vi "ROI from INI Section.vi"(7 "section":string="Parameters", 8 "error in (no error)":errorcluster, 11 "refnum in":T1) -> (0 "error out":errorcluster, 2 "ROI":T2 {"Contours"."Type" items=["No Selection", "Point", "Line", "Rectangle", "Oval", "Polygon", "Freehand Region", "Annulus", "Unused2", "Unused3", "Broken Line", "Freehand Line", "Rotated Rectangle"]}, 3 "refnum out":T1)   [LabVIEW 2020, in "POLARIS Vision utility.lvlib"]
uses:
  POLARIS Vision utility.lvlib
  <vilib>/Utility/config.llb/Config Data RefNum.ctl
  <vilib>/Utility/config.llb/Read Key (I32).vi
  <vilib>/Utility/config.llb/NI_LVConfig.lvlib
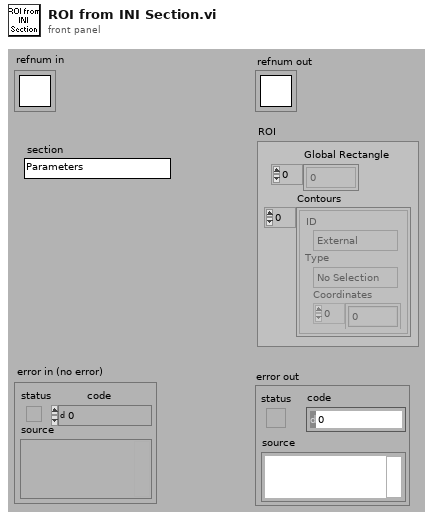
[diagram p1: front panel]
types:
  T1 = typedef "NI_LVConfig.lvlib/Config Data RefNum.ctl" = refnum<k1>
  T2 = typedef "ROI Descriptor" = cluster{"Global Rectangle":i32[], "Contours":cluster{"ID":enum32{"External", "Internal"}, "Type":u32, "Coordinates":i32[]}[]}
  T3 = cluster{"ID":enum32{"External", "Internal"}, "Type":u32, "Coordinates":i32[]}[]
  T4 = cluster{"ID":enum32{"External", "Internal"}, "Type":u32, "Coordinates":i32[]}
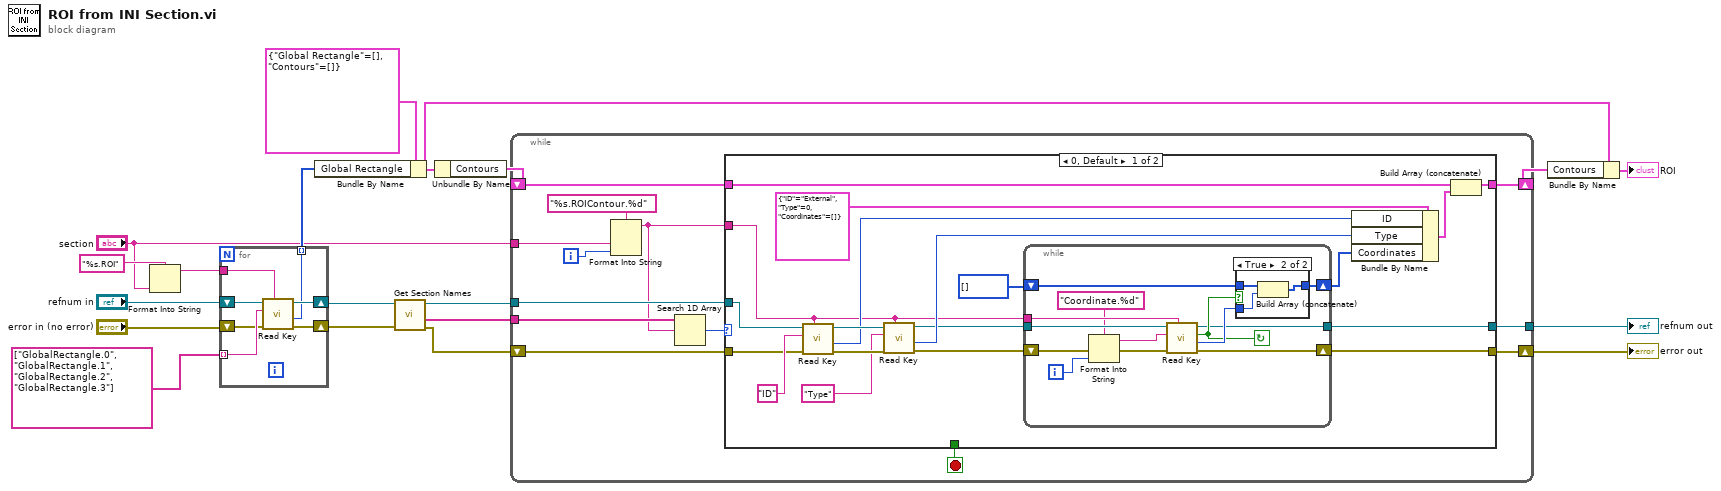
[diagram p0: block diagram]
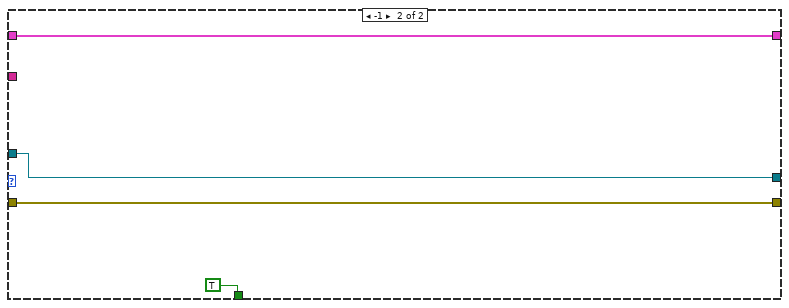
[diagram p3: hidden frame]
diagram:
  n1 = Format Into String(format string="%s.ROI", "section") -> (resulting string=w2:string)  [unwired: 2 in, 1 out]
  n2 = for {
    tunnel: string[] ["GlobalRectangle.0", "GlobalRectangle.1", "GlobalRectangle.2", "GlobalRectangle.3"] -> [w25] mode=indexing
    shift-right: [w24] -> w6
    shift-left: "refnum in" -> [w26]
    shift-right: [w22] -> w7
    shift-left: "error in (no error)" -> [w23]
    tunnel: [w21] -> w14 mode=indexing
    tunnel: w2 -> [w20]
    n3 = call-poly <vilib>:"Read Key.vi"("section"=w20, "error in (no error)"=w23, "key"=w25, "refnum"=w26) -> ("error out"=w22:errorcluster, "value"=w21:i32, "refnum out"=w24:T1)  [unwired: 4 in, 1 out]
  }
  n4 = Bundle By Name(cluster=T2 {"Global Rectangle"=[], "Contours"=[]} ("ROI Descriptor"), "Global Rectangle"=w14) -> (w12:T2)
  n5 = call <vilib>:"Get Section Names.vi"("error in (no error)"=w7, "refnum"=w6) -> ("error out"=w4:errorcluster, "section names"=w13:string[], "refnum out"=w5:T1)  [unwired: 7 in]
  n6 = Unbundle By Name(w12) -> ("Contours"=w17:T3)
  n7 = while {
    tunnel: w13 -> [w38]
    tunnel: w5 -> [w35]
    shift-right: [w33] -> w18
    shift-left: w4 -> [w34]
    tunnel: [w32] -> w19
    shift-right: [w30] -> w11
    shift-left: w17 -> [w31]
    tunnel: "section" -> [w28]
    i -> [w29]
    stop <- w36 stop-if-true
    n8 = Format Into String(format string="%s.ROIContour.%d" ("section"), w28, w29) -> (resulting string=w27:string)  [unwired: 2 in, 1 out]
    n9 = Search 1D Array(1D array=w38, element=w27) -> (index of element=w37:i32)  [unwired: 1 in]
    n10 = case shown="0, Default" w37 {
      tunnel: [_ TRUE] -> w36
      tunnel: w27 -> [w47 _]
      tunnel: w35 -> [w57 w77]
      tunnel: w34 -> [w56 w78]
      tunnel: w31 -> [w41 w76]
      tunnel: [w45 w78] -> w33
      tunnel: [w44 w77] -> w32
      tunnel: [w40 w76] -> w30
      frame 0, Default {
        n11 = call-poly <vilib>:"Read Key.vi"("section"=w47, "error in (no error)"=w56, "key"="ID", "refnum"=w57) -> ("error out"=w55:errorcluster, "value"=w51:i32, "refnum out"=w54:T1)  [unwired: 4 in, 1 out]
        n12 = call-poly <vilib>:"Read Key.vi"("section"=w47, "error in (no error)"=w55, "key"="Type", "refnum"=w54) -> ("error out"=w49:errorcluster, "value"=w50:i32, "refnum out"=w48:T1)  [unwired: 4 in, 1 out]
        n13 = while {
          tunnel: w48 -> [w70]
          tunnel: w47 -> [w71]
          shift-right: [w67] -> w43
          shift-left: i32[] [] ("Coordinates") -> [w69]
          shift-right: [w65] -> w45
          shift-left: w49 -> [w60]
          tunnel: [w64] -> w44
          i -> [w62]
          stop <- w66 continue-if-true
          n14 = Format Into String(format string="Coordinate.%d" ("string"), error in=w60, w62) -> (resulting string=w61:string, error out=w59:errorcluster)  [unwired: 1 in]
          n15 = call-poly <vilib>:"Read Key.vi"("section"=w71, "error in (no error)"=w59, "key"=w61, "refnum"=w70) -> ("error out"=w65:errorcluster, "value"=w68:i32, "found?"=w66:bool, "refnum out"=w64:T1)  [unwired: 4 in]
          n16 = case shown="True" w66 {
            tunnel: w69 -> [w72 w75]
            tunnel: w68 -> [_ w74]
            tunnel: [w72 w73] -> w67
            frame False {
            }
            frame True {
              n17 = Build Array (concatenate)(w75, w74) -> (w73:i32[])
            }
          }
        }
        n18 = Bundle By Name(cluster=T4 {"ID"=enum."External", "Type"=0, "Coordinates"=[]} ("element"), "ID"=w51, "Type"=w50, "Coordinates"=w43) -> (w42:T4)
        n19 = Build Array (concatenate)(w41, w42) -> (w40:T3)
      }
      frame -1 {
      }
    }
  }
  "error out" <- w18
  "refnum out" <- w19
  n20 = Bundle By Name(cluster=w12, "Contours"=w11) -> (→"ROI":T2)
